vi "7. System-Level Module.vi"() -> ()   [LabVIEW 2017]
doc: "### 7. System-Level Module.vi\n\n#### Overview\n\nDemonstrates how to create a system-level module and illustrates the differences between system-level and regular CSM modules when listing all active modules. System-level modules are typically used in large-scale projects to facilitate code development and debugging.\n\n#### Introduction\n\nThis example demonstrates how to create a system-level module and illustrates the differences between system-level and regular CSM modules when listing all active modules. System-level modules are typically used in large-scale projects to facilitate code development and debugging.\n\n#### Steps\n\nStep 1: Use high-level API VI to create a system-level module name (add \".\" as prefix to the CSM name to mark as system-level module). You can also just directly input the corresponding name string and rule symbols without calling this API if you're familiar with the rules.\n\nStep 2: Synchronized call of several \"normal\"/ non-System-level CSM modules.\n\nStep 3: Naming check of valid CSM module names, otherwise error will be generated. A valid CSM module name is a string which should NOT contain any of following special characters ~!@%^&*()\\[\\]{}+=|\\\\/?'\"<>,\\t\\r\\n, because those are reserved keywords for other well-defined purposes inside CSM framework. For further details you can go to another example code named Module Naming Rules.vi.\n\nStep 4: List all active CSM modules, by default no system-level modules will be listed. By using this high-level VI we can separate the system-level modules from other regular modules for better code development, debugging and so on.\n\nStep 5: Use high-level API VI under CSM->API->Non-CSM Caller Support to send synchronous Macro:Exit messages to all the active CSM modules to stop all those modules/VIs.\n\nThese Non-CSM Caller Support VIs are recommended to be used if we want to send inter-modules messages from a Non-CSM module to CSM-modules.\n\n#### Overview\n\nDemonstrates how to dynamically interact with CSM module attributes using VIs from outside the CSM framework.\n\n#### Introduction\n\nThis example demonstrates how to dynamically interact with CSM module attributes using VIs from outside the CSM framework.\n\nThe following are three ways of interaction within CSM framework:\n\n- Use string message queue to transfer message locally/outside of CSM framework, such as State >> Argument -@ DestModuleName.\n- Broadcast/Interrupt a status change event from a CSM module, register/unregister that event from another CSM/non-CSM module.\n- Use Module Attribute related VIs to get/set/remove/list CSM module attributes.\n\nThe core function of this example is from outside the CSM module to dynamically set another random number value to the CSM module, and then get the value from the CSM module and display the value on the UI.\n\n#### Steps\n\nStep 1: Drop the VI template from LabVIEW CSM palette.\n\nStep 2: Add one new line of state string after Macro:Initialize, namely API: Define ABC Attribute.\n\nStep 3: Set Module Attribute inside the CSM module: abc as attribute, a random number as value.\n\nStep 4: Set Module Attribute from outside the CSM module: abc as attribute, a random number as value.\n\nStep 5: Set Module Attribute from outside the CSM module: abc as attribute, retrieve the set random number as value.\n\nStep 6: Send a synchronous message to stop the CSM module from outside the CSM module."
uses:
  user.lib/_NEVSTOP/Communicable State Machine(CSM)/_Support/Error/CSM Invalid Name Error.vi
  user.lib/_NEVSTOP/Communicable State Machine(CSM)/Communicable State Machine.lvlib
panel:
  out "Module Names":string[](array[string])
  out "error out":errorcluster
  out "CSM Name(marked as Sysetem-Level Module)":string
  # "#CSM-Example Overview\n\nDemonstrates how to dynamically interact with CSM module attributes using VIs from outside the CSM framework."
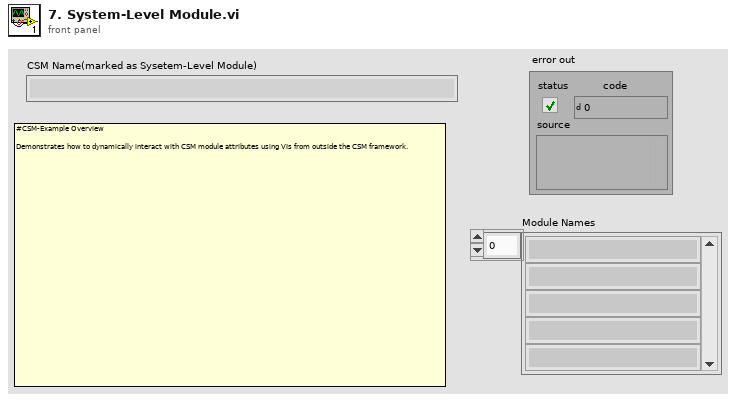
[diagram p1: front panel]
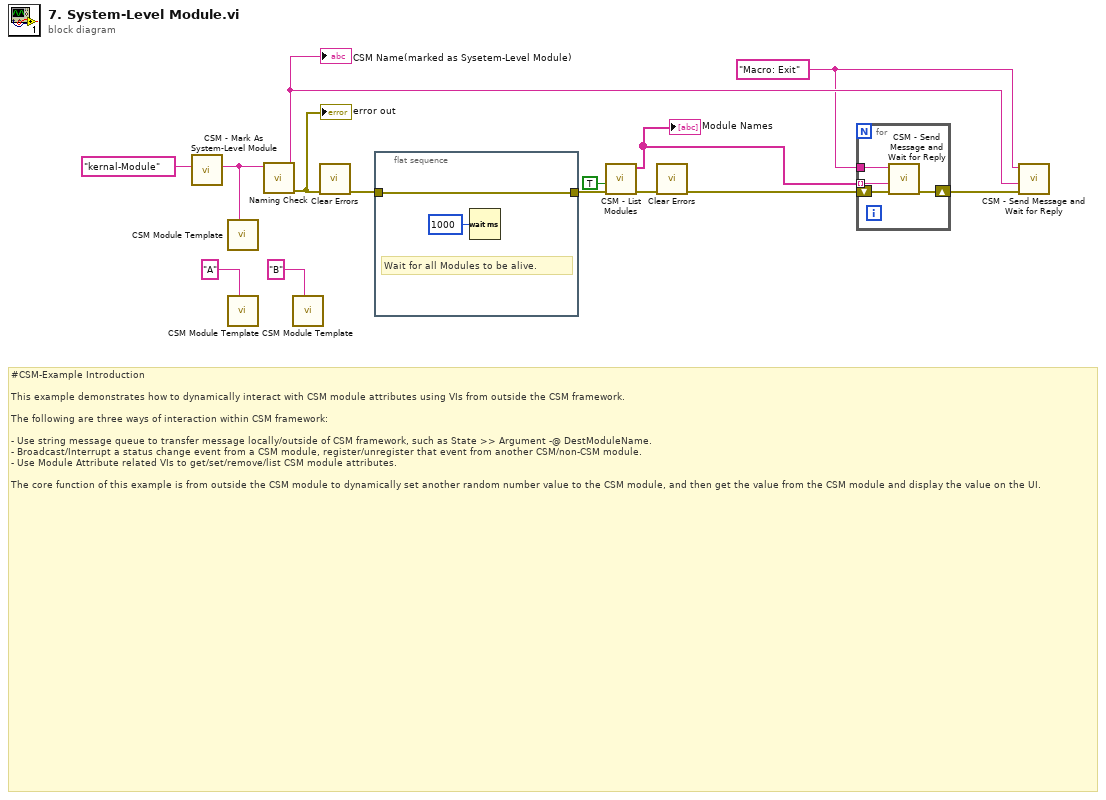
[diagram p0: block diagram]
diagram:
  w2 = "Macro: Exit" ("CSM Name")
  # "#CSM-Example Introduction\n\nThis example demonstrates how to dynamically interact with CSM module attributes using VIs from outside the CSM framework.\n\nThe following are three ways of interaction within CSM framework:\n\n- Use string message queue to transfer message locally/outside of CSM framework, such as State >> Argument -@ DestModuleName.\n- Broadcast/Interrupt a status change event from a CSM module, register/unregister that event from another CSM/non-CSM module.\n- Use Module Attribute related VIs to get/set/remove/list CSM module attributes.\n\nThe core function of this example is from outside the CSM module to dynamically set another random number value to the CSM module, and then get the value from the CSM module and display the value on the UI."
  n1 = call "CSM - Mark As System-Level Module.vi"("CSM Name"="kernal-Module") -> ("CSM Name (Marked As Sysetem-Level Module)"=w13:string)  [unwired: 9 in]
  n2 = call "CSM Module Template.vi"("Name (\"\" to Use UUID)"=w13) -> ()  [unwired: 11 in]
  n3 = call "CSM Module Template.vi"("Name (\"\" to Use UUID)"="A" ("Name(\"\" to use uuid)")) -> ()  [unwired: 11 in]
  n4 = call "Naming Check.vi"("Name (\"\" to Use UUID)"=w13) -> ("error out"=w12:errorcluster, "Name (Dup)"=w8:string)  [unwired: 9 in]
  "CSM Name(marked as Sysetem-Level Module)" <- w8
  "error out" <- w12
  n5 = call "CSM Module Template.vi"("Name (\"\" to Use UUID)"="B" ("Name(\"\" to use uuid)")) -> ()  [unwired: 11 in]
  n6 = call <vilib>:"Clear Errors.vi"("error in (no error)"=w12) -> ("error out"=w10:errorcluster)  [unwired: 5 in, 1 out]
  n7 = flat-sequence {
    tunnel: [w15] -> w11
    tunnel: w10 -> [w15]
    frame #0 {
      # "Wait for all Modules to be alive."
      n8 = Wait (ms)(milliseconds to wait=u32 1000) -> ()  [unwired: 1 out]
    }
  }
  n9 = call "CSM - List Modules.vi"("Error In"=w11, "With Instance? (F)"=TRUE ("All?")) -> ("error out"=w9:errorcluster, "Module Names"=w1:string[])  [unwired: 8 in]
  "Module Names" <- w1
  n10 = call <vilib>:"Clear Errors.vi"("error in (no error)"=w9) -> ("error out"=w6:errorcluster)  [unwired: 5 in, 1 out]
  n11 = for {
    tunnel: w2 -> [w18]
    shift-right: [w19] -> w5
    shift-left: w6 -> [w20]
    tunnel: w1 -> [w17] mode=indexing
    n12 = call "CSM - Send Message and Wait for Reply.vi"("Error In (No Error)"=w20, "Target Module"=w17, "State"=w18) -> ("error out"=w19:errorcluster)  [unwired: 6 in, 2 out]
  }
  n13 = call "CSM - Send Message and Wait for Reply.vi"("Error In (No Error)"=w5, "Target Module"=w8, "State"=w2) -> ()  [unwired: 6 in, 3 out]
